vi "SRV_PM_Search for Array Subset (U8).vi"(0 "1D Array":u8[](array[numeric]) format="%.0x", 7 "Search":u8[](array[numeric]) format="%.0x") -> (4 "Before Match":u8[](array[numeric]) format="%.0x", 6 "Match":u8[](array[numeric]) format="%.0x", 8 "After Match":u8[](array[numeric]) format="%.0x", 10 "Offset of Match":i32, 14 "Found?":bool, 15 "Offset After Match":i32)   [LabVIEW 2014]
doc: "Searches for Search array in 1D Array.\n\n\nAuthor: Mike Schultz"
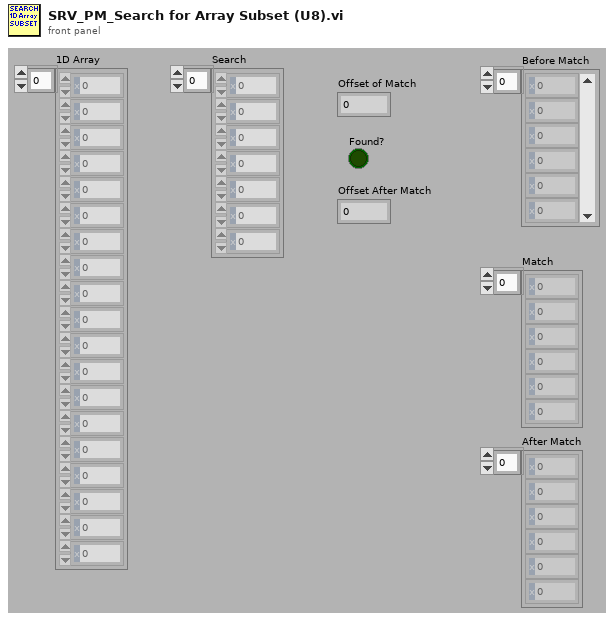
[diagram p1: front panel]
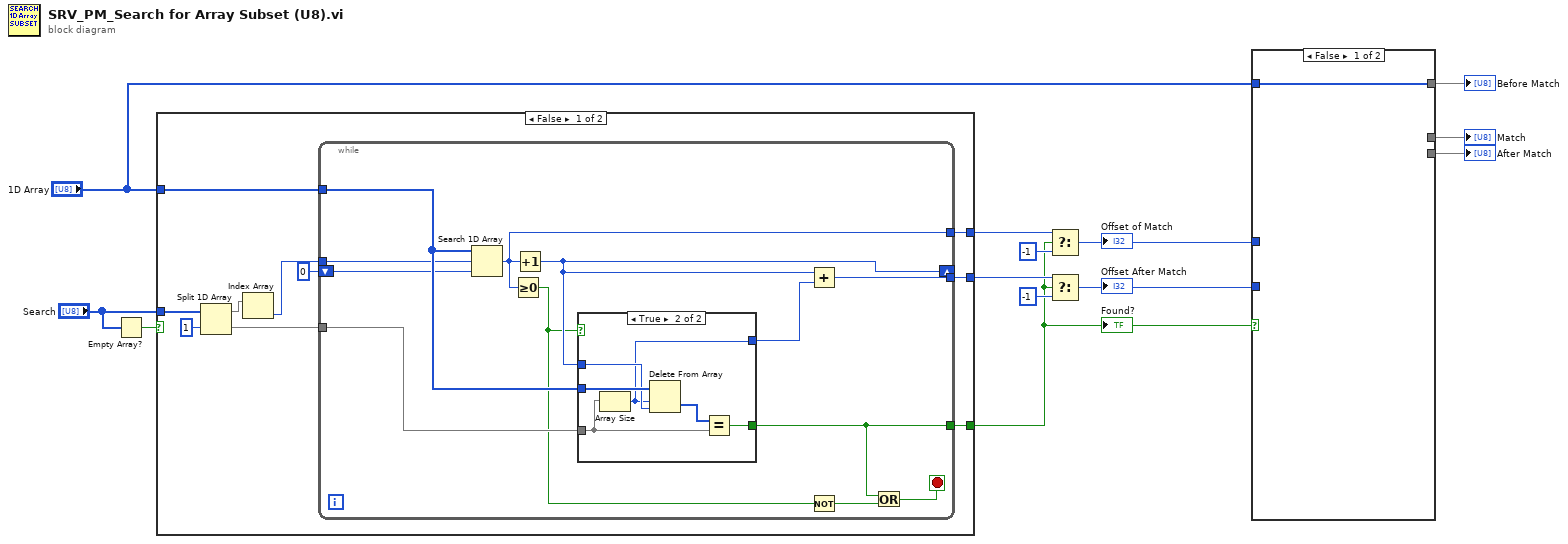
[diagram p0: block diagram]
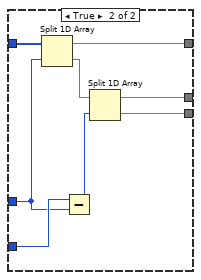
[diagram p2: hidden frame]
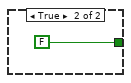
[diagram p4: hidden frame]
diagram:
  n1 = Empty Array?(array="Search") -> (empty?=w8:bool)
  n2 = case shown="False" w8 {
    tunnel: "1D Array" -> [w23 _]
    tunnel: [w22 _] -> w11
    tunnel: [w21 FALSE] -> w7
    tunnel: [w20 _] -> w10
    tunnel: "Search" -> [w17 _]
    frame False {
      n3 = Split 1D Array(array=w17, index=1) -> (first subarray=w14:u8[], second subarray=w16:u8[])
      n4 = Index Array(array=w14) -> (element=w15:u8)  [unwired: 1 in]
      n5 = while {
        tunnel: w23 -> [w35]
        tunnel: [w31] -> w22
        tunnel: [w24] -> w21
        tunnel: [w33] -> w20
        shift-right: [w28] -> _
        shift-left: 0 ("index of element") -> [w32]
        tunnel: w16 -> [w30]
        tunnel: w15 -> [w29]
        stop <- w26 stop-if-true
        n6 = Search 1D Array(1D array=w35, element=w29, start index (0)=w32) -> (index of element=w31:i32)
        n7 = Greater Or Equal To 0?(x=w31) -> (x >= 0?=w25:bool)
        n8 = Increment(x=w31) -> (x+1=w28:i32)
        n9 = case shown="True" w25 {
          selector: w25 -> [w36 _]
          tunnel: w35 -> [_ w42]
          tunnel: w30 -> [_ w40]
          tunnel: w28 -> [_ w41]
          tunnel: [w36 w38] -> w24
          tunnel: [_ w37] -> w34
          frame False {
          }
          frame True {
            n10 = Array Size(array=w40) -> (size(s)=w37:i32)
            n11 = Delete From Array(array=w42, length=w37, index=w41) -> (deleted portion=w39:u8[])  [unwired: 1 out]
            n12 = Equal?(x=w39, y=w40) -> (x = y?=w38:bool)
          }
        }
        n13 = Add(x=w28, y=w34) -> (x+y=w33:i32)
        n14 = Not(x=w25) -> (.not. x?=w27:bool)
        n15 = Or(x=w24, y=w27) -> (x .or. y?=w26:bool)
      }
    }
    frame True {
    }
  }
  "Found?" <- w7
  n16 = Select(t=w11, s=w7, f=-1) -> (s? t:f=w4:i32)
  "Offset of Match" <- w4
  n17 = Select(t=w10, s=w7, f=-1) -> (s? t:f=w3:i32)
  "Offset After Match" <- w3
  n18 = case shown="False" w7 {
    tunnel: "1D Array" -> [w44 w52]
    tunnel: [w44 w51] -> w5
    tunnel: w4 -> [_ w48]
    tunnel: w3 -> [_ w49]
    tunnel: [_ w46] -> w2
    tunnel: [_ w45] -> w1
    frame False {
    }
    frame True {
      n19 = Split 1D Array(array=w52, index=w48) -> (first subarray=w51:u8[], second subarray=w50:u8[])
      n20 = Subtract(x=w49, y=w48) -> (x-y=w47:i32)
      n21 = Split 1D Array(array=w50, index=w47) -> (first subarray=w46:u8[], second subarray=w45:u8[])
    }
  }
  "After Match" <- w1
  "Before Match" <- w5
  "Match" <- w2
